vi "AlliGator Load Single Gate Image from SS1 Dataset.vi"(6 "Action":T1, 8 "error in (no error)":errorcluster, 10 "File Info":variant, 11 "Gate Index":i32) -> (0 "error out":errorcluster, 1 "Data 2":sgl[][](array[numeric]), 3 "Data 1":sgl[][](array[numeric]))   [LabVIEW 2021, in "AlliGator Files.lvlib"]
doc: "Loads single gate image from SS1 dataset."
uses:
  AlliGator Files.lvlib
  AlliGator FLI Image Stack Action.ctl
  SwissSPAD/SwissSPAD 1 Extended Dataset Information.ctl
  SwissSPAD/SwissSPAD1 File Information.ctl
  SwissSPAD/SwissSPAD.lvlib
  AlliGator HDF5.lvlib
panel:
  # "see the AlliGator License on the block diagram (Ctrl+E or Window:Show Block Diagram)"
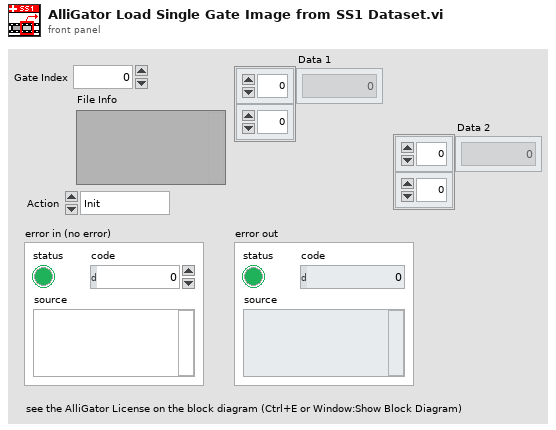
[diagram p1: front panel]
types:
  T1 = typedef "AlliGator HDF5.lvlib/AlliGator FLI Image Stack Action.ctl" = enum16{"Init", "Get Image", "Close"}
  T2 = typedef "SwissSPAD.lvlib/SwissSPAD 1 Extended Dataset Information.ctl" = cluster{"File Path":path, "Data Offset (in bytes)":i64, "# Bytes/Pixel":i32, "# Pixel X":i32, "# Pixel Y":i32, "SwissSPAD1 File Information":T3}
  T3 = typedef "SwissSPAD.lvlib/SwissSPAD1 File Information.ctl" = cluster{"SPAD Off Pattern":u64, "Recharge Pattern":u64, "Gate Pattern":u64, "Pattern Length":u32, "# Repetitions":u32, "Initial Macro Shift":u32, "Initial Micro Shift":u32, "VOP Voltage":dbl, "Top Gate Voltage":dbl, "Bias Voltage":dbl, "# Readouts/Frame":u32, "Scan Start (step unit)":u32, "Scan Increment (step unit)":u32, "# Frames":u32, "Note":string}
  T4 = enum16{"open", "replace", "create", "open or create", "replace or create", "replace or create with confirmation"}
  T5 = enum16{"big-endian, network order", "native, host order", "little-endian"}
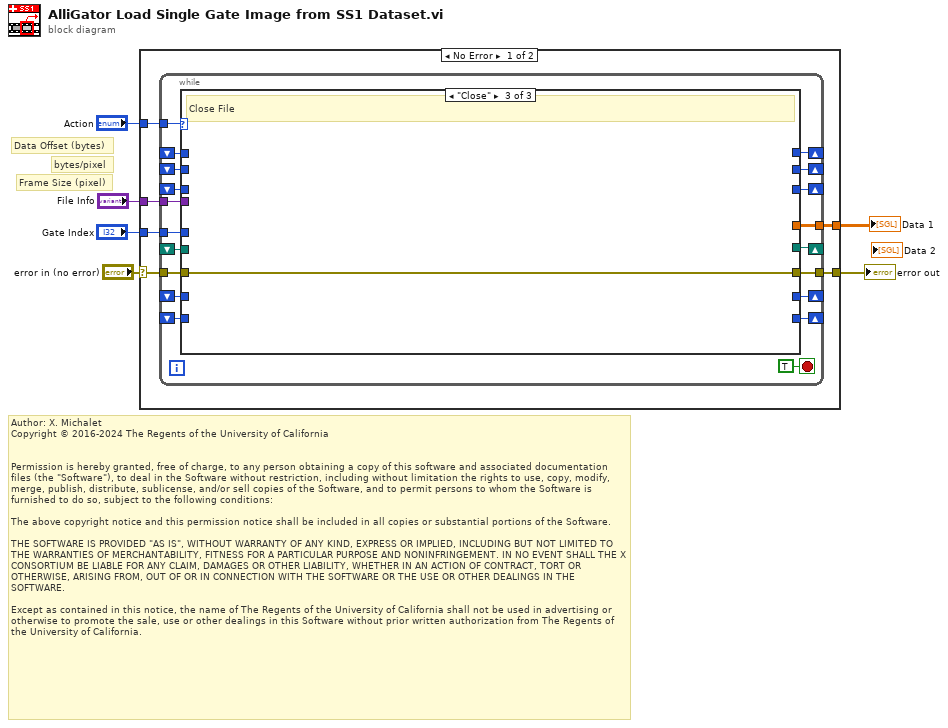
[diagram p0: block diagram]
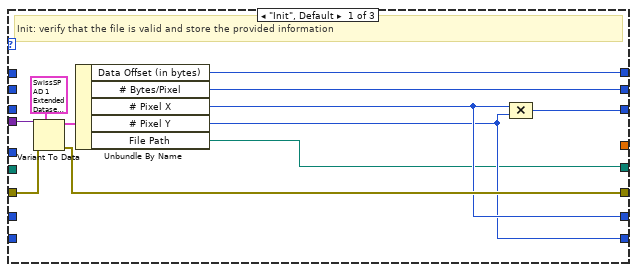
[diagram p2: hidden frame]
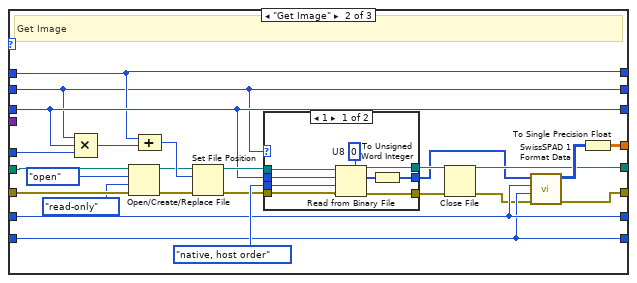
[diagram p3: hidden frame]
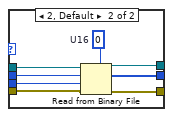
[diagram p4: hidden frame]
diagram:
  # "Author: X. Michalet\nCopyright © 2016-2024 The Regents of the University of California\n \n\nPermission is hereby granted, free of charge, to any person obtaining a copy of this software and associated documentation files (the \"Software\"), to deal in the Software without restriction, including without limitation the rights to use, copy, modify, merge, publish, distribute, sublicense, and/or sell copies of the Software, and to permit persons to whom the Software is furnished to do so, subject to the following conditions:\n\nThe above copyright notice and this permission notice shall be included in all copies or substantial portions of the Software.\n\nTHE SOFTWARE IS PROVIDED \"AS IS\", WITHOUT WARRANTY OF ANY KIND, EXPRESS OR IMPLIED, INCLUDING BUT NOT LIMITED TO THE WARRANTIES OF MERCHANTABILITY, FITNESS FOR A PARTICULAR PURPOSE AND NONINFRINGEMENT. IN NO EVENT SHALL THE X CONSORTIUM BE LIABLE FOR ANY CLAIM, DAMAGES OR OTHER LIABILITY, WHETHER IN AN ACTION OF CONTRACT, TORT OR OTHERWISE, ARISING FROM, OUT OF OR IN CONNECTION WITH THE SOFTWARE OR THE USE OR OTHER DEALINGS IN THE SOFTWARE.\n\nExcept as contained in this notice, the name of The Regents of the University of California shall not be used in advertising or otherwise to promote the sale, use or other dealings in this Software without prior written authorization from The Regents of the University of California."
  # "bytes/pixel"
  # "Frame Size (pixel)"
  # "Data Offset (bytes)"
  n1 = case shown="No Error" "error in (no error)" {
    selector: "error in (no error)" -> [w11 w86]
    tunnel: [w10 w86] -> w5
    tunnel: "Action" -> [w12 _]
    tunnel: "File Info" -> [w9 _]
    tunnel: "Gate Index" -> [w8 _]
    tunnel: [w7 _] -> w1
    frame No Error {
      n2 = while {
        tunnel: w12 -> [w30]
        tunnel: w11 -> [w29]
        tunnel: [w28] -> w10
        tunnel: w9 -> [w27]
        tunnel: w8 -> [w26]
        tunnel: [w25] -> w7
        shift-right: [w24] -> _
        shift-left: _ -> [w19]
        shift-right: [w23] -> _
        shift-left: _ -> [w18]
        shift-right: [w22] -> _
        shift-left: _ -> [w17]
        shift-right: [w21] -> _
        shift-left: _ -> [w20]
        shift-right: [w16] -> _
        shift-left: _ -> [w14]
        shift-right: [w15] -> _
        shift-left: _ -> [w13]
        stop <- TRUE stop-if-true
        n3 = case shown="\"Close\"" w30 {
          tunnel: w29 -> [w41 w64 w85]
          tunnel: [w36 w65 w85] -> w28
          tunnel: w27 -> [w42 _ _]
          tunnel: w26 -> [_ w44 _]
          tunnel: [_ w66 _] -> w25
          tunnel: [w38 w55 _] -> w24
          tunnel: [w33 w57 _] -> w23
          tunnel: [w37 w43 _] -> w22
          tunnel: [w32 w49 _] -> w21
          tunnel: w20 -> [_ w47 _]
          tunnel: w19 -> [_ w55 _]
          tunnel: w18 -> [_ w57 _]
          tunnel: w17 -> [_ w43 _]
          tunnel: [w35 w61 _] -> w16
          tunnel: [w34 w60 _] -> w15
          tunnel: w14 -> [_ w61 _]
          tunnel: w13 -> [_ w60 _]
          frame "Init", Default {
            # "Init: verify that the file is valid and store the provided information"
            n4 = Variant To Data(error in=w41, type=T2 {"File Path"=path "", "Data Offset (in bytes)"=0, "# Bytes/Pixel"=0, "# Pixel X"=0, "# Pixel Y"=0, "SwissSPAD1 File Information"={"SPAD Off Pattern"=0, "Recharge Pattern"=0, "Gate Pattern"=0, "Pattern Length"=0, "# Repetitions"=0, "Initial Macro Shift"=0, "Initial Micro Shift"=0, "VOP Voltage"=0.0, "Top Gate Voltage"=0.0, "Bias Voltage"=0.0, "# Readouts/Frame"=0, "Scan Start (step unit)"=0, "Scan Increment (step unit)"=0, "# Frames"=0, "Note"=""}} ("output cluster"), Variant=w42) -> (data=w39:T2, error out=w36:errorcluster)
            n5 = Unbundle By Name(w39) -> ("Data Offset (in bytes)"=w38:i64, "# Bytes/Pixel"=w37:i32, "# Pixel X"=w35:i32, "# Pixel Y"=w34:i32, "File Path"=w32:path)
            n6 = Compound Arithmetic op=MULTIPLY(w35, w34) -> (w33:i32)
          }
          frame "Get Image" {
            # "Get Image"
            n7 = Compound Arithmetic op=MULTIPLY(w43, w57, w44) -> (w56:i32)
            n8 = Open/Create/Replace File(file path (use dialog)=w47, error in=w64, operation (0:open)=T4."open", access (0:read/write)=enum16{"read/write", "read-only", "write-only"}."read-only") -> (refnum out=w52:refnum<file>, error out=w53:errorcluster)  [unwired: 2 in, 1 out]
            n9 = Compound Arithmetic op=ADD(w55, w56) -> (w54:i64)
            n10 = Set File Position(offset (in bytes) (0)=w54, refnum=w52, error in=w53) -> (refnum out=w58:refnum<file>, error out=w59:errorcluster)  [unwired: 1 in]
            n11 = case shown="1" w43 {
              tunnel: w58 -> [w76 w84]
              tunnel: [w75 w83] -> w50
              tunnel: w59 -> [w74 w82]
              tunnel: [w73 w81] -> w63
              tunnel: T5."native, host order" ("byte order (0:big-endian, network order)") -> [w72 w80]
              tunnel: w57 -> [w71 w77]
              tunnel: [w68 w78] -> w48
              frame 1 {
                w70 = u8 0  # U8
                n12 = Read from Binary File(5:w70, 8:w74, 9:w72, 10:w71, 11:w76) -> (0:w73:errorcluster, 2:w69:u8[], 3:w75:refnum<file>)  [unwired: 1 in, 1 out]
                n13 = To Unsigned Word Integer(number=w69) -> (unsigned 16bit integer=w68:u16[])
              }
              frame 2, Default {
                w79 = u16 0  # U16
                n14 = Read from Binary File(5:w79, 8:w82, 9:w80, 10:w77, 11:w84) -> (0:w81:errorcluster, 2:w78:u16[], 3:w83:refnum<file>)  [unwired: 1 in, 1 out]
              }
            }
            n15 = Close File(refnum=w50, error in=w63) -> (path=w49:path, error out=w51:errorcluster)
            n16 = call "SwissSPAD 1 Format Data.vi"("Error In"=w51, "Y Resolution"=w60, "X Resolution"=w61, "Flattened Image"=w48) -> ("Error Out"=w65:errorcluster, "Image out"=w67:u16[][])  [unwired: 6 in]
            n17 = To Single Precision Float(number=w67) -> (single precision float=w66:sgl[][])
          }
          frame "Close" {
            # "Close File"
          }
        }
      }
    }
    frame Error {
    }
  }
  "Data 1" <- w1
  "error out" <- w5
